vi "estruturas_dados_array.vi"() -> ()   [LabVIEW 2013]
panel:
  out "Array 2":dbl[][](array[numeric])
  out "Array":dbl[](array[numeric])
  out "Todas as Salas":string
  out "String 2":string
  out "Sala 1":string
  out "Sala 0":string
  in  "Salas":string[](array[string])
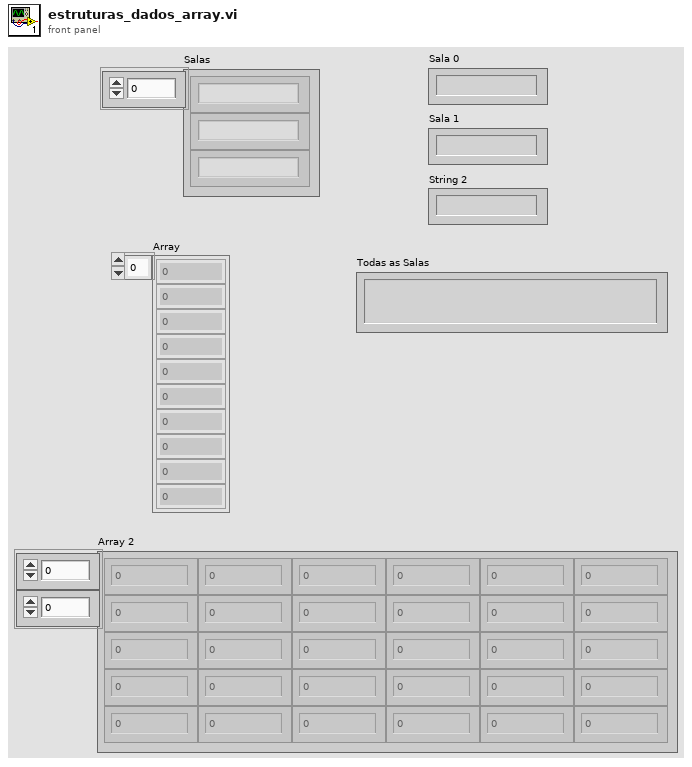
[diagram p1: front panel]
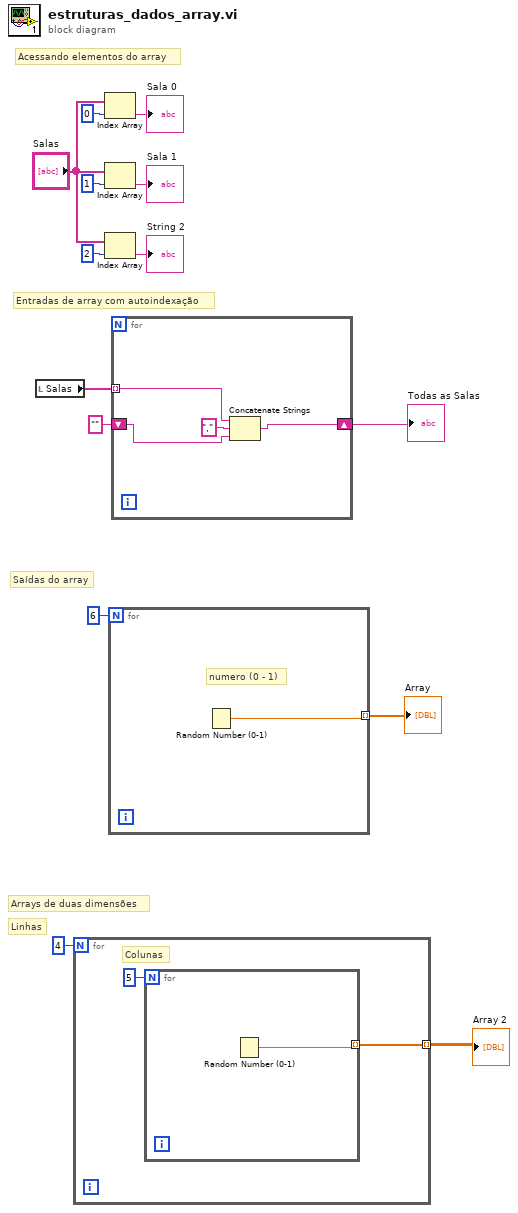
[diagram p0: block diagram]
diagram:
  # "Linhas"
  # "Arrays de duas dimensões"
  # "Saídas do array"
  # "Acessando elementos do array"
  # "Entradas de array com autoindexação"
  n1 = local read "Salas"() -> (w7:string[])
  n2 = for {
    N: 4 -> [_]
    tunnel: [w16] -> w1 mode=indexing
    # "Colunas"
    n3 = for {
      N: 5 -> [_]
      tunnel: [w17] -> w16 mode=indexing
      n4 = Random Number (0-1)() -> (number: 0 to 1=w17:dbl)
    }
  }
  "Array 2" <- w1
  n5 = Index Array(array="Salas", index=0) -> (element=→"Sala 0":string)
  n6 = Index Array(array="Salas", index=1) -> (element=→"Sala 1":string)
  n7 = Index Array(array="Salas", index=2) -> (element=→"String 2":string)
  n8 = for {
    N: 6 -> [_]
    tunnel: [w18] -> w3 mode=indexing
    # "numero (0 - 1)"
    n9 = Random Number (0-1)() -> (number: 0 to 1=w18:dbl)
  }
  "Array" <- w3
  n10 = for {
    tunnel: w7 -> [w22] mode=indexing
    shift-right: [w21] -> w6
    shift-left: "" -> [w19]
    n11 = Concatenate Strings(w22, "," ("string"), w19) -> (w21:string)
  }
  "Todas as Salas" <- w6
